vi "Get Attribute Type.vi"(7 "Test Executive Builder Data Type Handler in":refnum<class "Test Executive Builder Data Type Handler.lvclass">, 8 "error in (no error)":errorcluster, 11 "Potential Attribute in":variant) -> (0 "error out":errorcluster, 1 "Valid Type?":bool, 2 "Attribute Type":string, 3 "Potential Attribute out":variant)   [LabVIEW 2017, in "Test Executive Builder Data Type Handler.lvclass"]
uses:
  <vilib>/gpm_packages/@cs/Test-executive-builder/Source/Data Type Handler/Test Executive Builder Data Type Handler.lvclass
  <vilib>/gpm_packages/@cs/Test-executive-builder/Source/Test Executive Builder Dialogs/String Type View/String Type View.lvclass
  <vilib>/gpm_packages/@cs/Test-executive-builder/Source/Test Executive Builder Dialogs/Integer Type View/Integer Type View.lvclass
  <vilib>/gpm_packages/@cs/Test-executive-builder/Source/Test Executive Builder Dialogs/Float Type View/Float Type View.lvclass
  <vilib>/gpm_packages/@cs/Test-executive-builder/Source/Test Executive Builder Dialogs/Boolean Type View/Boolean Type View.lvclass
  <vilib>/Utility/Data Type/NI_Data Type.lvlib
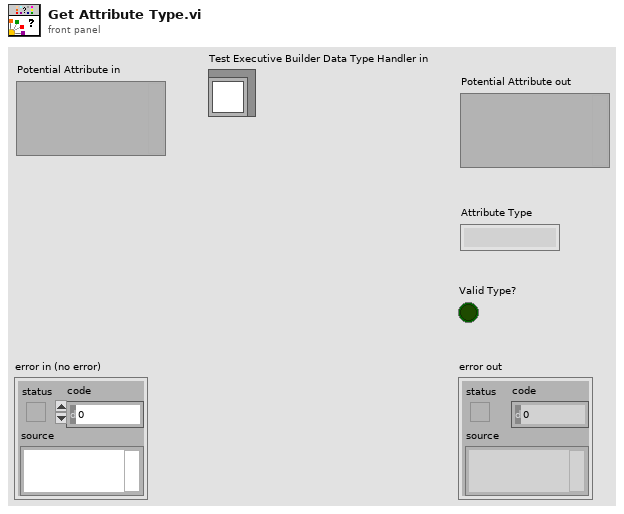
[diagram p1: front panel]
types:
  T1 = typedef "NI_Data Type.lvlib/Data Type.ctl" = enum8{"Invalid Type", "Void", "I8", "I16", "I32", "I64", "U8", "U16", "U32", "U64", "Single Float", "Double Float", "Extended Float", "Single Complex", "Double Complex", "Extended Complex", "Enum U8", "Enum U16", "Enum U32", "Enum U64", "Single Float With Unit", "Double Float With Unit", "Extended Float With Unit", "Single Complex with Unit", "Double Complex with Unit", "Extended Complex with Unit", "Boolean", "String", "Path", "Picture", "Tag", "Array", "Cluster", "Variant", "LV Variant", "Waveform", "Timestamp", "Digital Waveform", "Digital Data", "ExpressData", "Refnum", "External Data", "VI", "Poly VI", "LabVIEW Class Instance", "Fixed Point"}
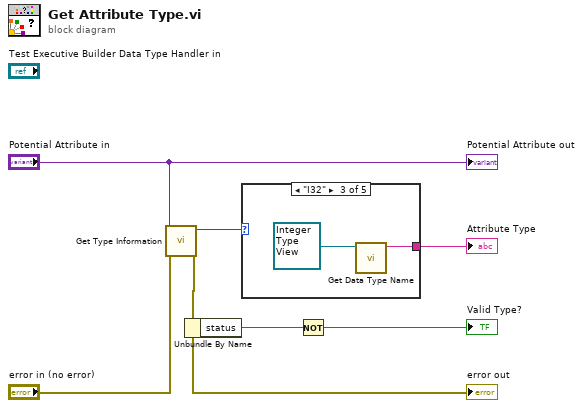
[diagram p0: block diagram]
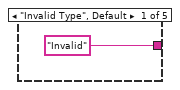
[diagram p2: hidden frame]
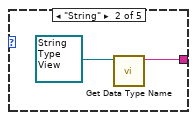
[diagram p3: hidden frame]
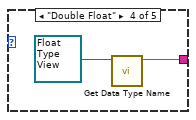
[diagram p4: hidden frame]
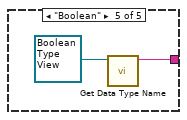
[diagram p5: hidden frame]
diagram:
  n1 = call <vilib>:"Get Type Information.vi"("error in (no error)"="error in (no error)", "Variant"="Potential Attribute in") -> ("error out"=w3:errorcluster, "Type"=w2:T1)  [unwired: 5 in, 3 out]
  "error out" <- w3
  n2 = Unbundle By Name(w3) -> ("status"=w7:bool)
  n3 = case shown="\"I32\"" w2 {
    tunnel: ["Invalid" ("Data Type Name") w9 w11 w13 w15] -> w1
    frame "Invalid Type", Default {
    }
    frame "String" {
      n4 = call-dynamic "Get Data Type Name.vi"("String Type View in"=refnum<class "String Type View.lvclass"> refnum ("String Type View.lvclass")) -> ("Data Type Name"=w9:string)  [unwired: 10 in]
    }
    frame "I32" {
      n5 = call-dynamic "Get Data Type Name.vi"("String Type View in"=refnum<class "Integer Type View.lvclass"> refnum ("Integer Type View.lvclass")) -> ("Data Type Name"=w11:string)  [unwired: 10 in]
    }
    frame "Double Float" {
      n6 = call-dynamic "Get Data Type Name.vi"("String Type View in"=refnum<class "Float Type View.lvclass"> refnum ("Float Type View.lvclass")) -> ("Data Type Name"=w13:string)  [unwired: 10 in]
    }
    frame "Boolean" {
      n7 = call-dynamic "Get Data Type Name.vi"("Boolean Type View in"=refnum<class "Boolean Type View.lvclass"> refnum ("Boolean Type View.lvclass")) -> ("Data Type Name"=w15:string)  [unwired: 10 in]
    }
  }
  "Attribute Type" <- w1
  n8 = Not(x=w7) -> (.not. x?=→"Valid Type?":bool)
  "Potential Attribute out" <- "Potential Attribute in"
